vi "Variant to Packed String.vi"(2 "Variant":variant) -> (4 "Type Descriptor":i16[](array[numeric]) format="%x", 5 "Packed String":string)   [LabVIEW 2018, in "Application.lvlib" / "Store.lvclass"]
uses:
  Store.lvclass
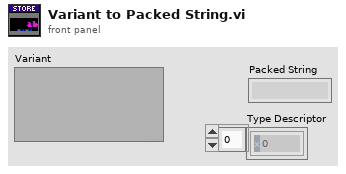
[diagram p1: front panel]
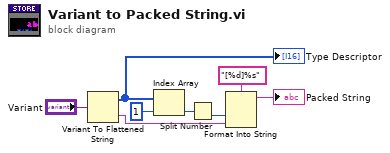
[diagram p0: block diagram]
diagram:
  n1 = Variant To Flattened String(Variant="Variant") -> (data string=w5:string, 1:w4:i16[])
  "Type Descriptor" <- w4
  n2 = Index Array(array=w4, index=1) -> (element=w7:i16)
  n3 = Split Number(x=w7) -> (lo(x)=w6:u8)  [unwired: 1 out]
  n4 = Format Into String(format string="[%d]%s", w6, w5) -> (resulting string=→"Packed String":string)  [unwired: 2 in, 1 out]
